vi "ukol2.vi"() -> ()   [LabVIEW 2023]
uses:
  <vilib>/Waveform/WDTOps.llb/WDT Get Final Time Value DBL.vi
  <vilib>/Waveform/WDTOps.llb/WDT Get Waveform Subset DBL.vi
panel:
  out "tf":timestamp
  out "Waveform Graph 2":waveform(dbl)(graph)
  out "Waveform Graph":waveform(dbl)[](graph)
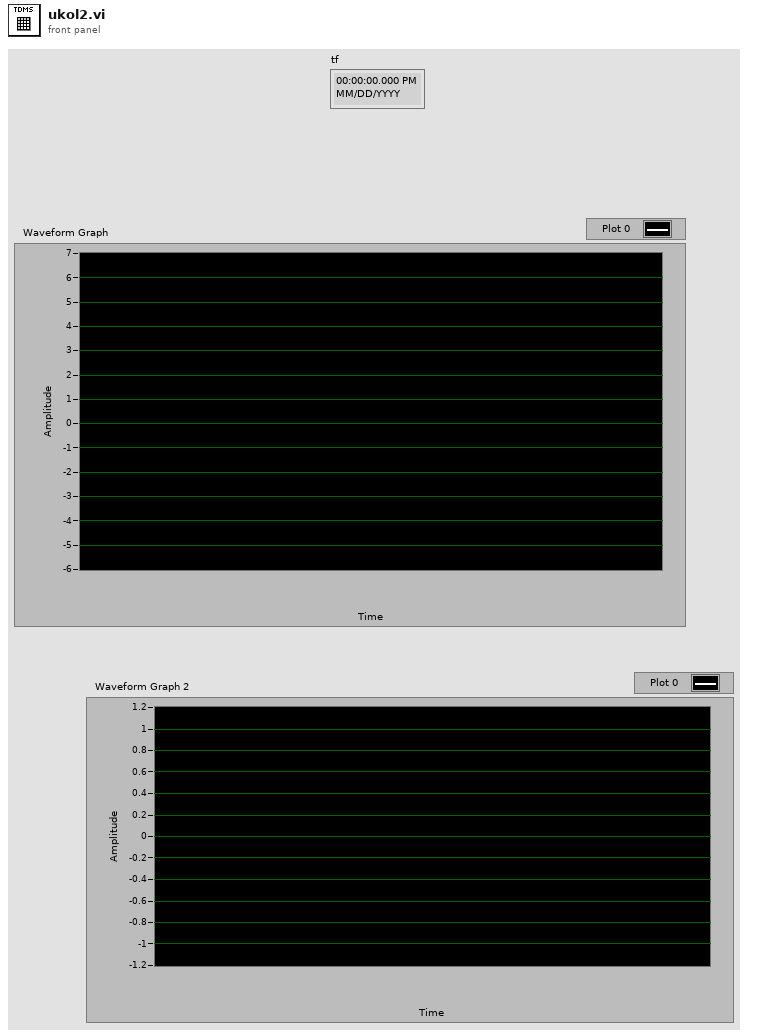
[diagram p1: front panel]
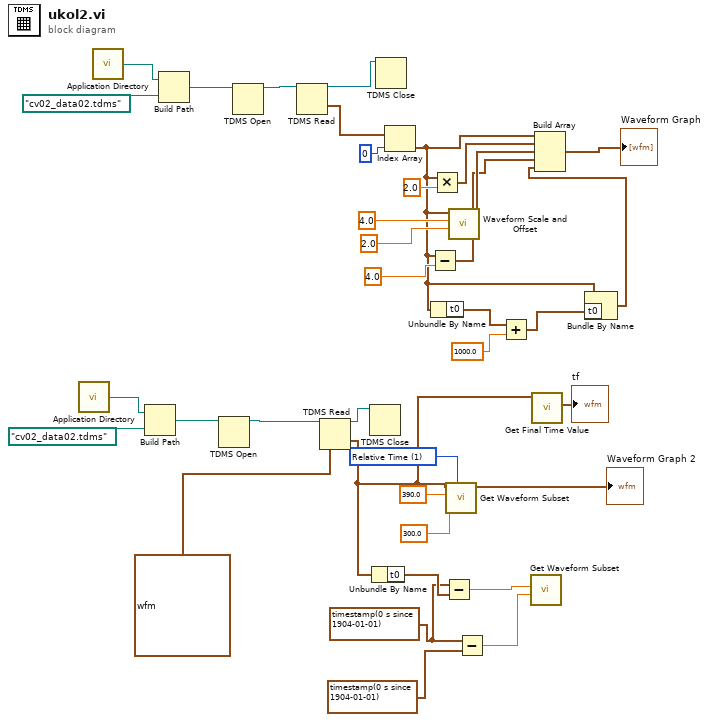
[diagram p0: block diagram]
diagram:
  w4 = timestamp(0 s since 1904-01-01) ("t0")
  w6 = u16 1 items=["Samples", "Relative Time"] ("start/duration format")
  n1 = call <vilib>:"Application Directory.vi"() -> ("Application Directory"=w20:path)
  n2 = call <vilib>:"Application Directory.vi"() -> ("Application Directory"=w27:path)
  n3 = Build Path(base path=w20, name or relative path=path "cv02_data02.tdms") -> (appended path=w18:path)
  n4 = Build Path(base path=w27, name or relative path=path "cv02_data02.tdms") -> (appended path=w25:path)
  n5 = TDMS Open(11:w18) -> (3:w17:refnum<k34>)  [unwired: 6 in, 1 out]
  n6 = TDMS Open(11:w25) -> (3:w23:refnum<k34>)  [unwired: 6 in, 1 out]
  n7 = TDMS Read(0:w23) -> (4:w37:refnum<k34>, 10:w36:waveform(dbl)[])  [unwired: 7 in, 4 out]
  n8 = TDMS Read(0:w17, 12:waveform(dbl) {"t0"=timestamp(0 s since 1904-01-01), "dt"=1.0, "Y"=[]} ("data type")) -> (4:w21:refnum<k34>, 10:w7:waveform(dbl))  [unwired: 6 in, 4 out]
  n9 = TDMS Close(11:w21) -> ()  [unwired: 1 in, 2 out]
  n10 = Unbundle By Name(w7) -> ("t0"=w5:timestamp)
  n11 = TDMS Close(11:w37) -> ()  [unwired: 1 in, 2 out]
  n12 = Index Array(array=w36, index=0) -> (element=w11:waveform(dbl))
  n13 = Subtract(x=w11, y=4.0) -> (x-y=w29:waveform(dbl))
  n14 = Unbundle By Name(w11) -> ("t0"=w10:timestamp)
  n15 = Multiply(x=w11, y=2.0) -> (x*y=w33:waveform(dbl))
  n16 = Subtract(x=w4, y=w5) -> (x-y=w2:dbl)
  n17 = call-poly <vilib>:"Get Waveform Subset.vi"("start/duration format"=w6, "duration"=300.0, "start samples/time"=390.0, "waveform in"=w7) -> ("waveform out"=→"Waveform Graph 2":waveform(dbl))  [unwired: 2 in, 3 out]
  n18 = call <vilib>:"Waveform Scale and Offset.vi"("scale"=2.0, "offset"=4.0, "waveform in"=w11) -> ("waveform out"=w31:waveform(dbl))  [unwired: 7 in, 1 out]
  n19 = Subtract(x=w4, y=timestamp(0 s since 1904-01-01) ("t0")) -> (x-y=w1:dbl)
  n20 = Add(x=w10, y=1000.0) -> (x+y=w9:timestamp)
  n21 = call-poly <vilib>:"Get Waveform Subset.vi"("duration"=w1, "start samples/time"=w2) -> ()  [unwired: 4 in, 4 out]
  n22 = call-poly <vilib>:"Get Final Time Value.vi"("waveform in"=w7) -> ("tf"=→"tf":timestamp)  [unwired: 8 in, 2 out]
  n23 = Bundle By Name(cluster=w11, "t0"=w9) -> (w12:waveform(dbl))
  n24 = Build Array(w11, w33, w31, w29, w12) -> (→"Waveform Graph":waveform(dbl)[])
